vi "InitialMap.vi"() -> (3 "Map":dbl[][](array[numeric]))   [LabVIEW 2011]
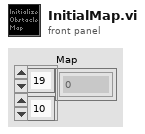
[diagram p1: front panel]
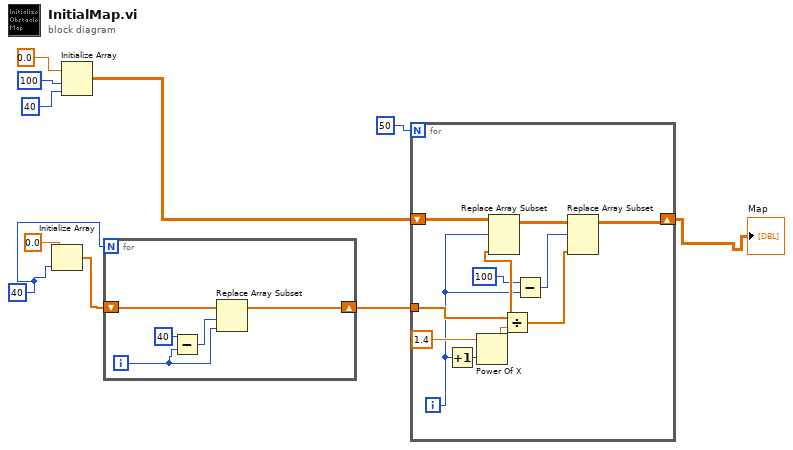
[diagram p0: block diagram]
diagram:
  w5 = 40 ("dimension size")
  n1 = Initialize Array(0.0 ("element"), w5) -> (w6:dbl[])
  n2 = Initialize Array(0.0 ("element"), 100 ("dimension size"), 40 ("dimension size")) -> (w4:dbl[][])
  n3 = for {
    N: w5 -> [_]
    shift-right: [w14] -> w3
    shift-left: w6 -> [w15]
    i -> [w12]
    n4 = Subtract(x=40, y=w12) -> (x-y=w11:i32)
    n5 = Replace Array Subset(array=w15, new element=w12, index=w11) -> (w14:dbl[])
  }
  n6 = for {
    N: 50 -> [_]
    shift-right: [w23] -> w1
    shift-left: w4 -> [w25]
    tunnel: w3 -> [w26]
    i -> [w17]
    n7 = Increment(x=w17) -> (x+1=w16:i32)
    n8 = Power Of X(1:w16, 2:1.4 ("y")) -> (0:w19:dbl)
    n9 = Divide(x=w26, y=w19) -> (x/y=w22:dbl[])
    n10 = Replace Array Subset(array=w25, new element=w22, index (row)=w17) -> (w24:dbl[][])  [unwired: 1 in]
    n11 = Subtract(x=100, y=w17) -> (x-y=w20:i32)
    n12 = Replace Array Subset(array=w24, new element=w22, index (row)=w20) -> (w23:dbl[][])  [unwired: 1 in]
  }
  "Map" <- w1
